vi "Nominal Value Write Array.vi"(0 "Current Nominal Value in":refnum<class "Current Nominal Value.lvclass">, 1 "Current Nominal Value Value":dbl[](array[numeric]), 3 "error in":errorcluster) -> (7 "Current Nominal Value out":refnum<class "Current Nominal Value.lvclass">, 10 "error out":errorcluster)   [LabVIEW 2023, in "Current Nominal Value.lvclass"]
uses:
  Current Nominal Value.lvclass
  Parents/Nominal Value/Nominal Value.lvclass
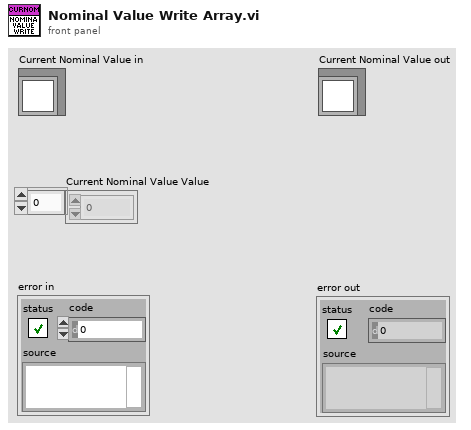
[diagram p1: front panel]
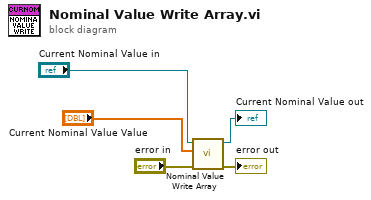
[diagram p0: block diagram]
diagram:
  n1 = call-parent "Nominal Value Write Array.vi"("Nominal Value in"="Current Nominal Value in", "Nominal Value Value"="Current Nominal Value Value", "error in"="error in") -> ("Nominal Value out"=→"Current Nominal Value out":refnum<class "Current Nominal Value.lvclass">, "error out"=→"error out":errorcluster)  [unwired: 6 in]
